vi "XNET Write.vi"   [LabVIEW 2025]
doc: "Writes data to the network using an XNET session."
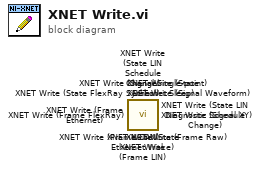
[diagram p0: block diagram]
diagram:
  n1 = call <vilib>:"XNET Write (State Ethernet Wake).vi"() -> ()  [unwired: 14 in, 2 out]
  n2 = call <vilib>:"XNET Write (State Ethernet Sleep).vi"() -> ()  [unwired: 14 in, 2 out]
  n3 = call <vilib>:"XNET Write (Frame Ethernet).vi"() -> ()  [unwired: 14 in, 2 out]
  n4 = call <vilib>:"XNET Write (State LIN Diagnostic Schedule Change).vi"() -> ()  [unwired: 14 in, 2 out]
  n5 = call <vilib>:"XNET Write (State FlexRay Symbol).vi"() -> ()  [unwired: 14 in, 2 out]
  n6 = call <vilib>:"XNET Write (State LIN Schedule Change).vi"() -> ()  [unwired: 14 in, 2 out]
  n7 = call <vilib>:"XNET Write (Frame LIN).vi"() -> ()  [unwired: 14 in, 2 out]
  n8 = call <vilib>:"XNET Write (Frame Raw).vi"() -> ()  [unwired: 14 in, 2 out]
  n9 = call <vilib>:"XNET Write (Frame FlexRay).vi"() -> ()  [unwired: 14 in, 2 out]
  n10 = call "XNET Write (Frame CAN).vi"() -> ()  [unwired: 14 in, 2 out]
  n11 = call <vilib>:"XNET Write (Signal XY).vi"() -> ()  [unwired: 14 in, 2 out]
  n12 = call <vilib>:"XNET Write (Signal Waveform) .vi"() -> ()  [unwired: 14 in, 2 out]
  n13 = call <vilib>:"XNET Write (Signal Single-point).vi"() -> ()  [unwired: 14 in, 2 out]
